vi "Get Temperature.vi"(8 "error in (no error)":errorcluster, 9 "ChipID":u32=65535 format="%x", 10 "LayerID":u32=65535 format="%x", 11 "connection ID":refnum<k5>) -> (0 "error out":errorcluster, 2 "Temperatures":u32[](array[numeric]) format="%x", 3 "connection ID out":refnum<k5>, 4 "Get Temperature done":string)   [LabVIEW 2015, in "VIPM2.lvlib"]
uses:
  VIPM2.lvlib
panel:
  out "Ready to receive parameters":string
  # "Get Temperature"
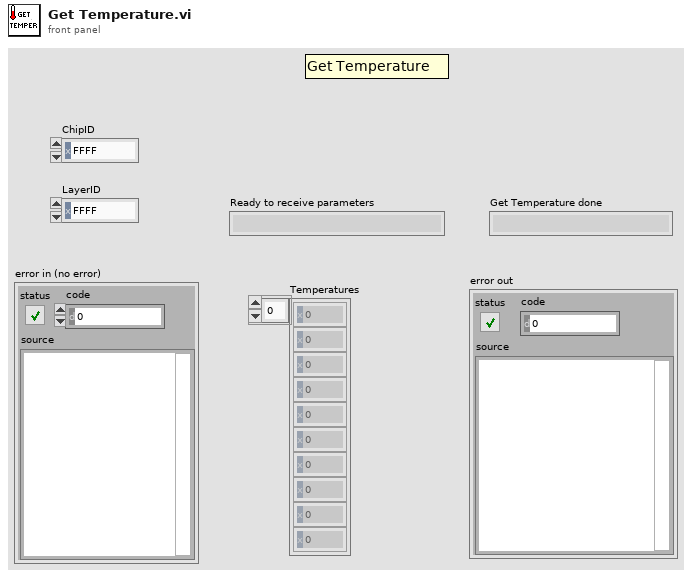
[diagram p1: front panel]
types:
  T1 = enum16{"Standard", "Buffered", "CRLF", "Immediate"}
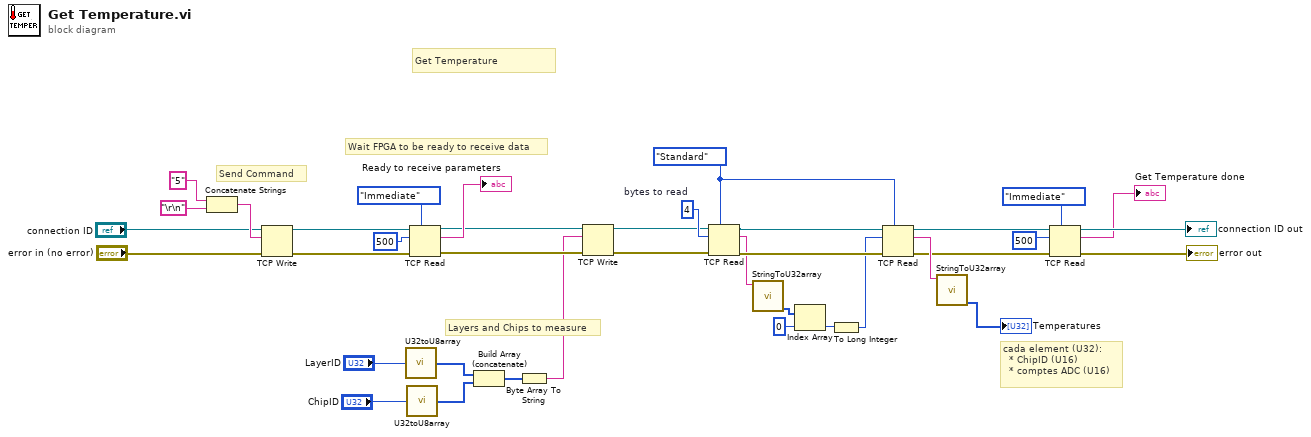
[diagram p0: block diagram]
diagram:
  w11 = 4  # bytes to read
  w12 = T1."Standard" ("mode (standard)")
  # "cada element (U32):\n  * ChipID (U16)\n  * comptes ADC (U16)"
  # "Layers and Chips to measure"
  # "Wait FPGA to be ready to receive data"
  # "Send Command"
  # "Get Temperature"
  n1 = Concatenate Strings("5" ("string"), "\r\n") -> (w36:string)
  n2 = TCP Write(connection ID="connection ID", data in=w36, error in (no error)="error in (no error)") -> (connection ID out=w30:refnum<k5>, error out=w29:errorcluster)  [unwired: 1 in, 1 out]
  n3 = call "U32toU8array.vi"("x"="LayerID") -> ("ArrayU8"=w18:u8[])
  n4 = call "U32toU8array.vi"("x"="ChipID") -> ("ArrayU8"=w16:u8[])
  n5 = TCP Read(connection ID=w30, bytes to read=500, error in (no error)=w29, 7:T1."Immediate" ("mode (standard)")) -> (connection ID out=w27:refnum<k5>, data out=→"Ready to receive parameters":string, error out=w26:errorcluster)  [unwired: 1 in]
  n6 = Build Array (concatenate)(w18, w16) -> (w19:u8[])
  n7 = Byte Array To String(unsigned byte array=w19) -> (string=w25:string)
  n8 = TCP Write(connection ID=w27, data in=w25, error in (no error)=w26) -> (connection ID out=w7:refnum<k5>, error out=w6:errorcluster)  [unwired: 1 in, 1 out]
  n9 = TCP Read(connection ID=w7, bytes to read=w11, error in (no error)=w6, 7:w12) -> (connection ID out=w15:refnum<k5>, data out=w10:string, error out=w14:errorcluster)  [unwired: 1 in]
  n10 = call "StringToU32array.vi"("String"=w10) -> ("U32array"=w9:u32[])  [unwired: 2 out]
  n11 = Index Array(array=w9, index=0) -> (element=w2:u32)
  n12 = To Long Integer(number=w2) -> (32bit integer=w1:i32)
  n13 = TCP Read(connection ID=w15, bytes to read=w1, error in (no error)=w14, 7:w12) -> (connection ID out=w5:refnum<k5>, data out=w8:string, error out=w4:errorcluster)  [unwired: 1 in]
  n14 = call "StringToU32array.vi"("String"=w8) -> ("U32array"=→"Temperatures":u32[])  [unwired: 2 out]
  n15 = TCP Read(connection ID=w5, bytes to read=500, error in (no error)=w4, 7:T1."Immediate" ("mode (standard)")) -> (connection ID out=→"connection ID out":refnum<k5>, data out=→"Get Temperature done":string, error out=→"error out":errorcluster)  [unwired: 1 in]
